vi "GitHash.vi"(10 "git repo path":path=path "C:/", 11 "git.exe path":path=path "C:/Program Files/Git/cmd/git.exe") -> (0 "error out":errorcluster, 1 "Fetch error?":bool, 2 "Resolved version":T1, 3 "Version string":string)   [LabVIEW 2012]
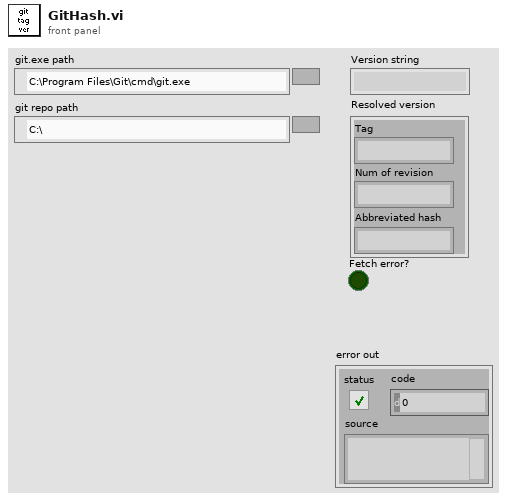
[diagram p1: front panel]
types:
  T1 = cluster{"Tag":string, "Num of revision":string, "Abbreviated hash":string}
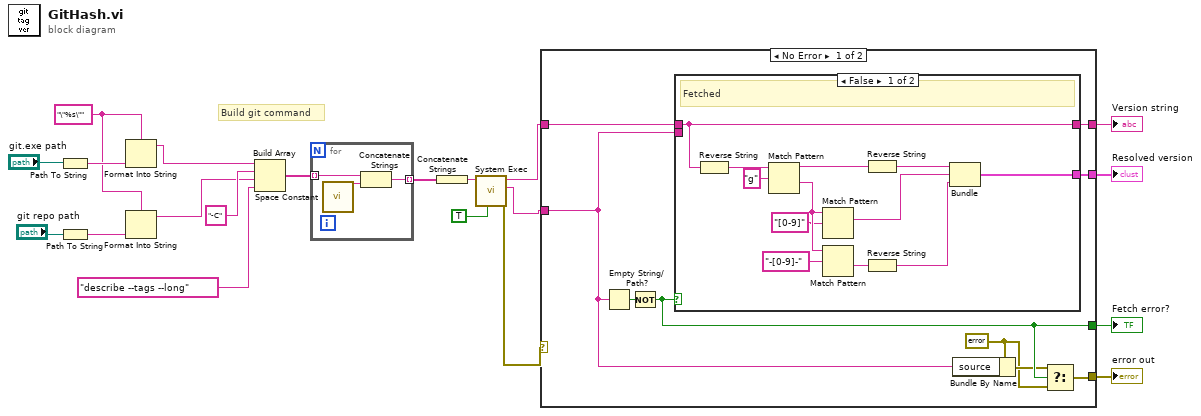
[diagram p0: block diagram]
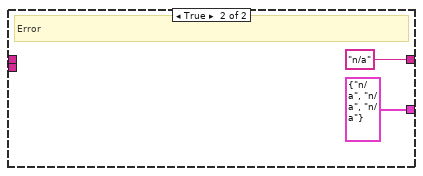
[diagram p2: hidden frame]
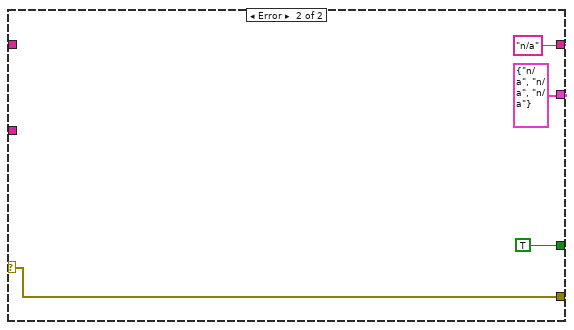
[diagram p3: hidden frame]
diagram:
  w6 = "\"%s\"" ("format string")
  # "Build git command"
  n1 = Path To String(path="git.exe path") -> (string=w7:string)
  n2 = Path To String(path="git repo path") -> (string=w5:string)
  n3 = Format Into String(format string=w6, w7) -> (resulting string=w4:string)  [unwired: 2 in, 1 out]
  n4 = Format Into String(format string=w6, w5) -> (resulting string=w3:string)  [unwired: 2 in, 1 out]
  n5 = Build Array(w4, "-C" ("string"), w3, "describe --tags --long" ("string")) -> (w9:string[])
  n6 = for {
    tunnel: w9 -> [w23] mode=indexing
    tunnel: [w21] -> w8 mode=indexing
    n7 = call <vilib>:"Space Constant.vi"() -> ("String"=w22:string)
    n8 = Concatenate Strings(w23, w22) -> (w21:string)
  }
  n9 = Concatenate Strings(w8) -> (w2:string)
  n10 = call <vilib>:"System Exec.vi"("run minimized? (F)"=TRUE, "command line"=w2) -> ("error out"=w14:errorcluster, "standard error"=w15:string, "standard output"=w16:string)  [unwired: 6 in, 1 out]
  n11 = case shown="No Error" w14 {
    selector: w14 -> [_ w47]
    tunnel: [w32 TRUE] -> w20
    tunnel: [w31 w47] -> w19
    tunnel: [w30 "n/a" ("standard output")] -> w18
    tunnel: [w29 cluster{string, string, string} {"n/a", "n/a", "n/a"}] -> w17
    tunnel: w16 -> [w26 _]
    tunnel: w15 -> [w25 _]
    frame No Error {
      w24 = errorcluster {"status"=FALSE, "code"=0, "source"=""} ("error in (no error)")
      n12 = Empty String/Path?(string/path=w25) -> (empty?=w28:bool)
      n13 = Not(x=w28) -> (.not. x?=w32:bool)
      n14 = case shown="False" w32 {
        tunnel: w26 -> [w37 _]
        tunnel: [w37 "n/a" ("standard output")] -> w30
        tunnel: [w33 cluster{string, string, string} {"n/a", "n/a", "n/a"}] -> w29
        tunnel: w25 -> [_ _]
        frame False {
          # "Fetched"
          n15 = Reverse String(1:w37) -> (0:w38:string)
          n16 = Match Pattern(string=w38, regular expression="g") -> (before substring=w40:string, after substring=w43:string)  [unwired: 1 in, 2 out]
          n17 = Match Pattern(string=w43, regular expression="[0-9]") -> (match substring=w35:string)  [unwired: 1 in, 3 out]
          n18 = Match Pattern(string=w43, regular expression="-[0-9]-") -> (after substring=w44:string)  [unwired: 1 in, 3 out]
          n19 = Reverse String(1:w40) -> (0:w36:string)
          n20 = Reverse String(1:w44) -> (0:w34:string)
          n21 = Bundle(w36, w35, w34) -> (w33:cluster{string, string, string})  [unwired: 1 in]
        }
        frame True {
          # "Error"
        }
      }
      n22 = Bundle By Name(cluster=w24, "source"=w25) -> (w27:errorcluster)
      n23 = Select(t=w27, s=w32, f=w24) -> (s? t:f=w31:errorcluster)
    }
    frame Error {
    }
  }
  "Fetch error?" <- w20
  "error out" <- w19
  "Version string" <- w18
  "Resolved version" <- w17
